vi "LoadMDF.vi"(1 "relative path":string) -> (0 "MDF":T2(array[cluster])=[{"Type"=enum."Start", "X"=100, "Y"=100, "Speed"=10, "Behaviors"=enum."Open Water Transit"}, {"Type"=enum."Waypoint", "X"=449, "Y"=569, "Speed"=4, "Behaviors"=enum."Open Water Transit"}, {"Type"=enum."Waypoint", "X"=803, "Y"=515, "Speed"=4, "Behaviors"=enum."Open Water Transit"}, {"Type"=enum."Waypoint", "X"=911, "Y"=689, "Speed"=4, "Behaviors"=enum."Open Water Transit"}, {"Type"=enum."Waypoint", "X"=755, "Y"=881, "Speed"=4, "Behaviors"=enum."Open Water Transit"}, {"Type"=enum."End", "X"=0, "Y"=0, "Speed"=0, "Behaviors"=enum."Open Water Transit"}])   [LabVIEW 2014]
uses:
  <vilib>/Utility/file.llb/Read From Spreadsheet File (string).vi
panel:
  in  "MDF seed":T1={"Type"=enum."Start", "X"=101, "Y"=0, "Speed"=0, "Behaviors"=enum."Open Water Transit"}
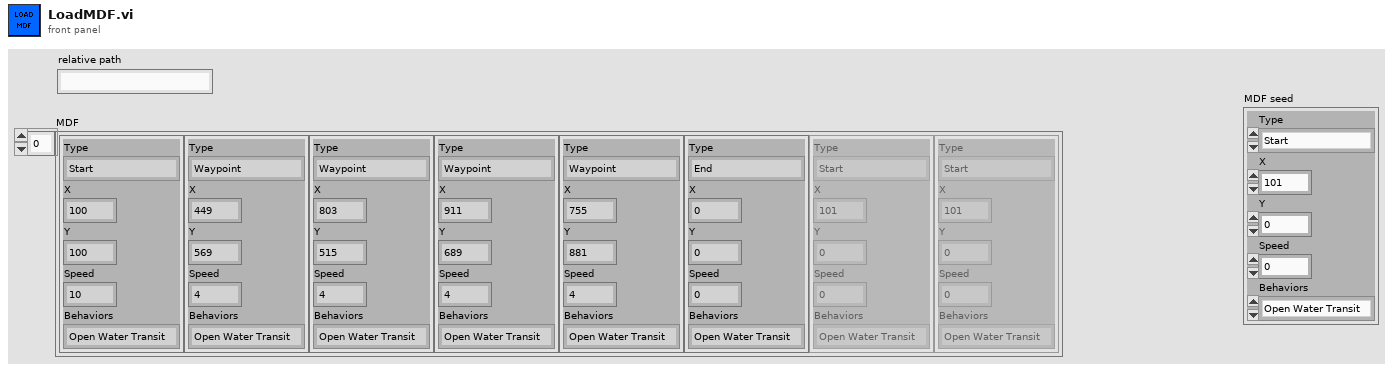
[diagram p1: front panel]
types:
  T1 = cluster{"Type":enum16{"Start", "Waypoint", "End"}, "X":i32, "Y":i32, "Speed":i32, "Behaviors":enum16{"Open Water Transit", "P-Wall Follow", "S-Wall Follow", "Dock"}}
  T2 = cluster{"Type":enum16{"Start", "Waypoint", "End"}, "X":i32, "Y":i32, "Speed":i32, "Behaviors":enum16{"Open Water Transit", "P-Wall Follow", "S-Wall Follow", "Dock"}}[]
  T3 = enum16{"Open Water Transit", "P-Wall Follow", "S-Wall Follow", "Dock"}
  T4 = cluster{"all rows[0]":string, "all rows[1]":string, "all rows[2]":string, "all rows[3]":string, "all rows[4]":string}
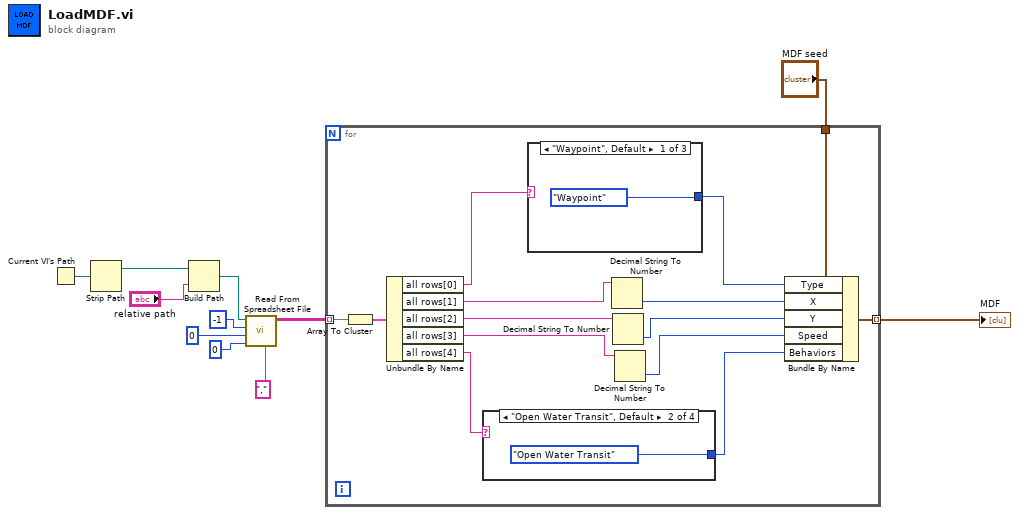
[diagram p0: block diagram]
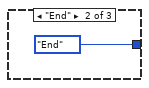
[diagram p2: hidden frame]
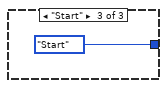
[diagram p3: hidden frame]
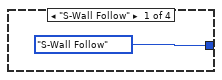
[diagram p4: hidden frame]
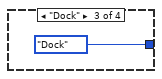
[diagram p5: hidden frame]
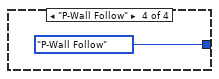
[diagram p6: hidden frame]
diagram:
  n1 = Current VI's Path() -> (path=w5:path)
  n2 = Strip Path(path=w5) -> (stripped path=w4:path)  [unwired: 1 out]
  n3 = Build Path(base path=w4, name or relative path="relative path") -> (appended path=w6:path)
  n4 = call-poly <vilib>:"Read From Spreadsheet File.vi"("delimiter (\\t)"="," ("delimiter (\\t)"), "max characters/row  (no limit:0)"=0, "start of read offset (chars.:0)"=0, "number of rows (all:-1)"=-1, "file path (dialog if empty)"=w6) -> ("all rows"=w3:string[][])  [unwired: 2 in, 4 out]
  n5 = for {
    tunnel: w3 -> [w25] mode=indexing
    tunnel: "MDF seed" -> [w23]
    tunnel: [w22] -> w1 mode=indexing
    n6 = Array To Cluster(array=w25) -> (cluster=w24:T4)
    n7 = Unbundle By Name(w24) -> ("all rows[0]"=w13:string, "all rows[1]"=w21:string, "all rows[2]"=w19:string, "all rows[3]"=w17:string, "all rows[4]"=w15:string)
    n8 = case shown="\"Open Water Transit\", Default" w15 {
      tunnel: [T3."S-Wall Follow" ("Behaviors") T3."Open Water Transit" ("Behaviors") T3."Dock" ("Behaviors") T3."P-Wall Follow" ("Behaviors")] -> w14
      frame "S-Wall Follow" {
      }
      frame "Open Water Transit", Default {
      }
      frame "Dock" {
      }
      frame "P-Wall Follow" {
      }
    }
    n9 = case shown="\"Waypoint\", Default" w13 {
      tunnel: [enum16{"Start", "Waypoint", "End"}."Waypoint" ("Type") enum16{"Start", "Waypoint", "End"}."End" ("Type") enum16{"Start", "Waypoint", "End"}."Start" ("Type")] -> w12
      frame "Waypoint", Default {
      }
      frame "End" {
      }
      frame "Start" {
      }
    }
    n10 = Decimal String To Number(string=w21) -> (number=w20:i32)  [unwired: 2 in, 1 out]
    n11 = Decimal String To Number(string=w19) -> (number=w18:i32)  [unwired: 2 in, 1 out]
    n12 = Decimal String To Number(string=w17) -> (number=w16:i32)  [unwired: 2 in, 1 out]
    n13 = Bundle By Name(cluster=w23, "Type"=w12, "X"=w20, "Y"=w18, "Speed"=w16, "Behaviors"=w14) -> (w22:T1)
  }
  "MDF" <- w1
